vi "Configure List Save Or Recall.vi"(8 "error in (no error)":errorcluster, 9 "File Name(1)":u8=1 min=1 max=10 step=1, 10 "SAVE OR REC  (SAVE)":bool=TRUE, 11 "VISA resource name":refnum<visa-resource-name>) -> (0 "error out":errorcluster, 3 "VISA resource name out":refnum<visa-resource-name>)   [LabVIEW 2020, in "IT6500.lvlib"]
doc: "This command is used to save or invoke the edited LIST file"
uses:
  IT6500.lvlib
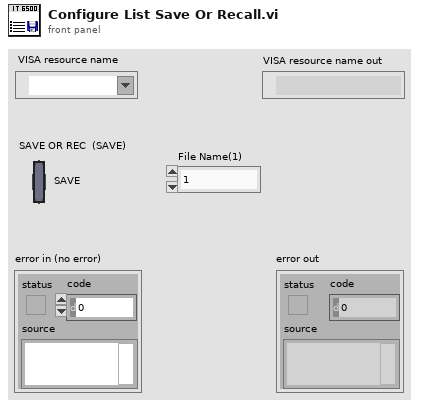
[diagram p1: front panel]
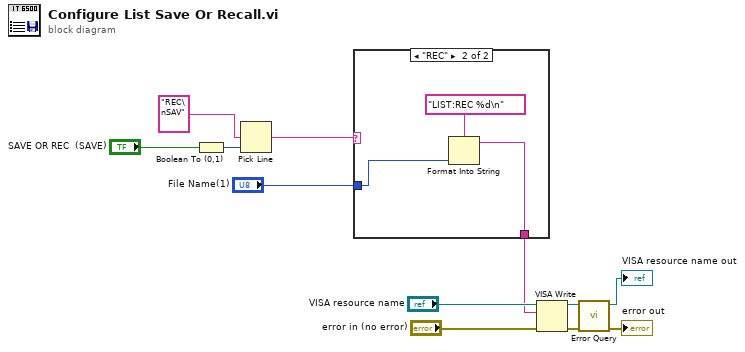
[diagram p0: block diagram]
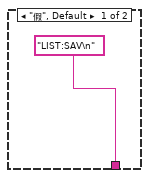
[diagram p2: hidden frame]
diagram:
  n1 = Boolean To (0,1)(Boolean="SAVE OR REC  (SAVE)") -> (0, 1=w5:i16)
  n2 = Pick Line(multi-line string="REC\nSAV", line index=w5) -> (output string=w2:string)  [unwired: 1 in]
  n3 = case shown="\"REC\"" w2 {
    tunnel: ["LIST:SAV\n" w15] -> w3
    tunnel: "File Name(1)" -> [_ w14]
    frame "假", Default {
    }
    frame "REC" {
      n4 = Format Into String(format string="LIST:REC %d\n", w14) -> (resulting string=w15:string)  [unwired: 2 in, 1 out]
    }
  }
  n5 = VISA Write(VISA resource name="VISA resource name", write buffer=w3, error in (no error)="error in (no error)") -> (VISA resource name out=w10:refnum<visa-resource-name>, error out=w9:errorcluster)  [unwired: 1 out]
  n6 = call "Error Query.vi"("error in (no error)"=w9, "VISA resource name"=w10) -> ("error out"=→"error out":errorcluster, "VISA resource name out"=→"VISA resource name out":refnum<visa-resource-name>)  [unwired: 6 in, 2 out]
